vi "XNET Read (State Session Info).vi"(0 "session in":refnum<k21>, 11 "error in (no error)":errorcluster) -> (4 "session out":refnum<k21>, 6 "session info state":T1 items=["Stopped", "Started", "Mix"], 15 "error out":errorcluster)   [LabVIEW 2018]
doc: "Reads the current state for the session."
uses:
  XNET Session Info State.ctl
  nixlvapi.dll
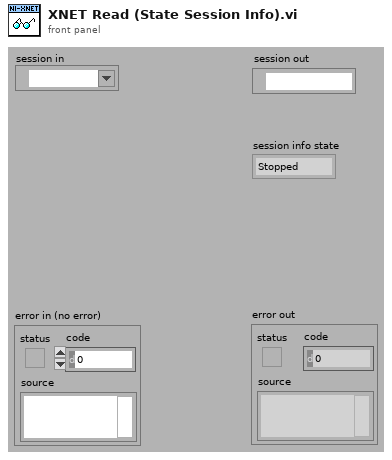
[diagram p1: front panel]
types:
  T1 = typedef "XNET Session Info State.ctl" = u8
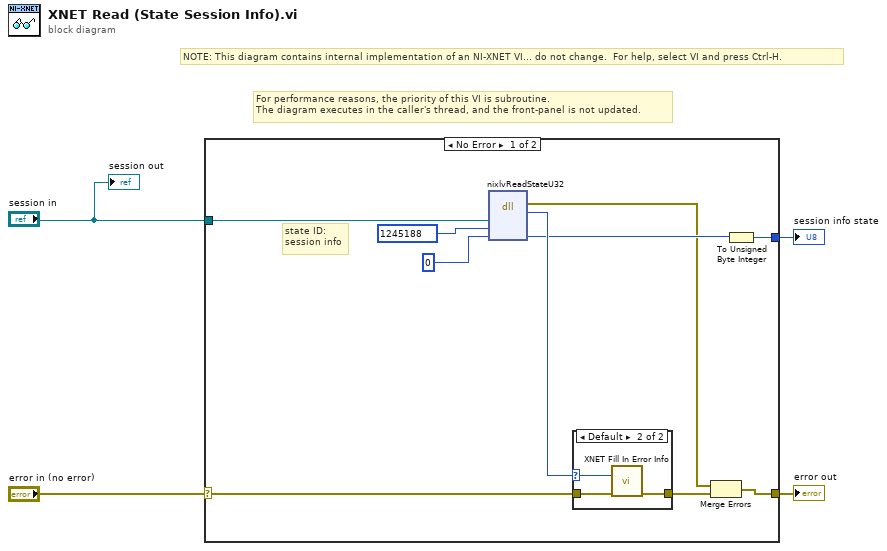
[diagram p0: block diagram]
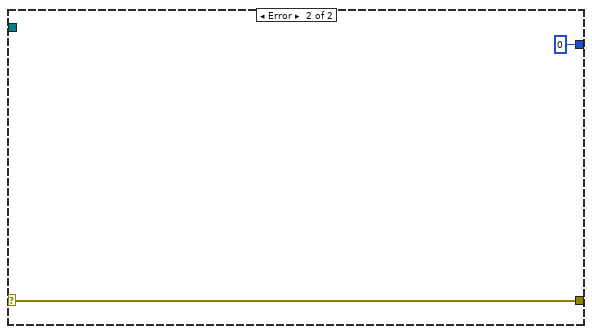
[diagram p3: hidden frame]
diagram:
  # "For performance reasons, the priority of this VI is subroutine.\nThe diagram executes in the caller's thread, and the front-panel is not updated."
  # "NOTE: This diagram contains internal implementation of an NI-XNET VI... do not change.  For help, select VI and press Ctrl-H."
  n1 = case shown="No Error" "error in (no error)" {
    selector: "error in (no error)" -> [w13 w20]
    tunnel: "session in" -> [w14 _]
    tunnel: [w6 w20] -> w4
    tunnel: [w8 u8 0] -> w1
    frame No Error {
      # "state ID: \nsession info"
      n2 = dll-call lib="nixlvapi.*" fn="nixlvReadStateU32"("sessionRef"=w14, "stateID"=u32 1245188 ("ParamOut"), "value"=u32 0) -> (error out=w5:errorcluster, "return type"=w11:i32, "value"=w9:u32)  [unwired: 4 in, 2 out]
      n3 = case shown="Default" w11 {
        selector: w11 -> [_ w16]
        tunnel: w13 -> [w15 w17]
        tunnel: [w15 w18] -> w12
        frame 0 {
        }
        frame Default {
          n4 = call "XNET Fill In Error Info.vi"("status code"=w16, "error in"=w17) -> ("error out"=w18:errorcluster)  [unwired: 13 out]
        }
      }
      n5 = Merge Errors(w5, w12) -> (w6:errorcluster)
      n6 = To Unsigned Byte Integer(number=w9) -> (unsigned 8bit integer=w8:u8)
    }
    frame Error {
    }
  }
  "error out" <- w4
  "session info state" <- w1
  "session out" <- "session in"
